vi "EnumDevicesByGenTL.vi"(0 "error in (no error)":errorcluster caption="错误输入（无错误）", 1 "pIFInfo":T2) -> (2 "error out":errorcluster caption="错误输出", 3 "function return":i32, 4 "nDeviceNum":u32, 5 "pGenTLDevInfoArray":T1(array[cluster]))   [LabVIEW 2013, in "MvCameraControl.lvlib"]
uses:
  MvCameraControl.lvlib
  MvCameraPatch.dll
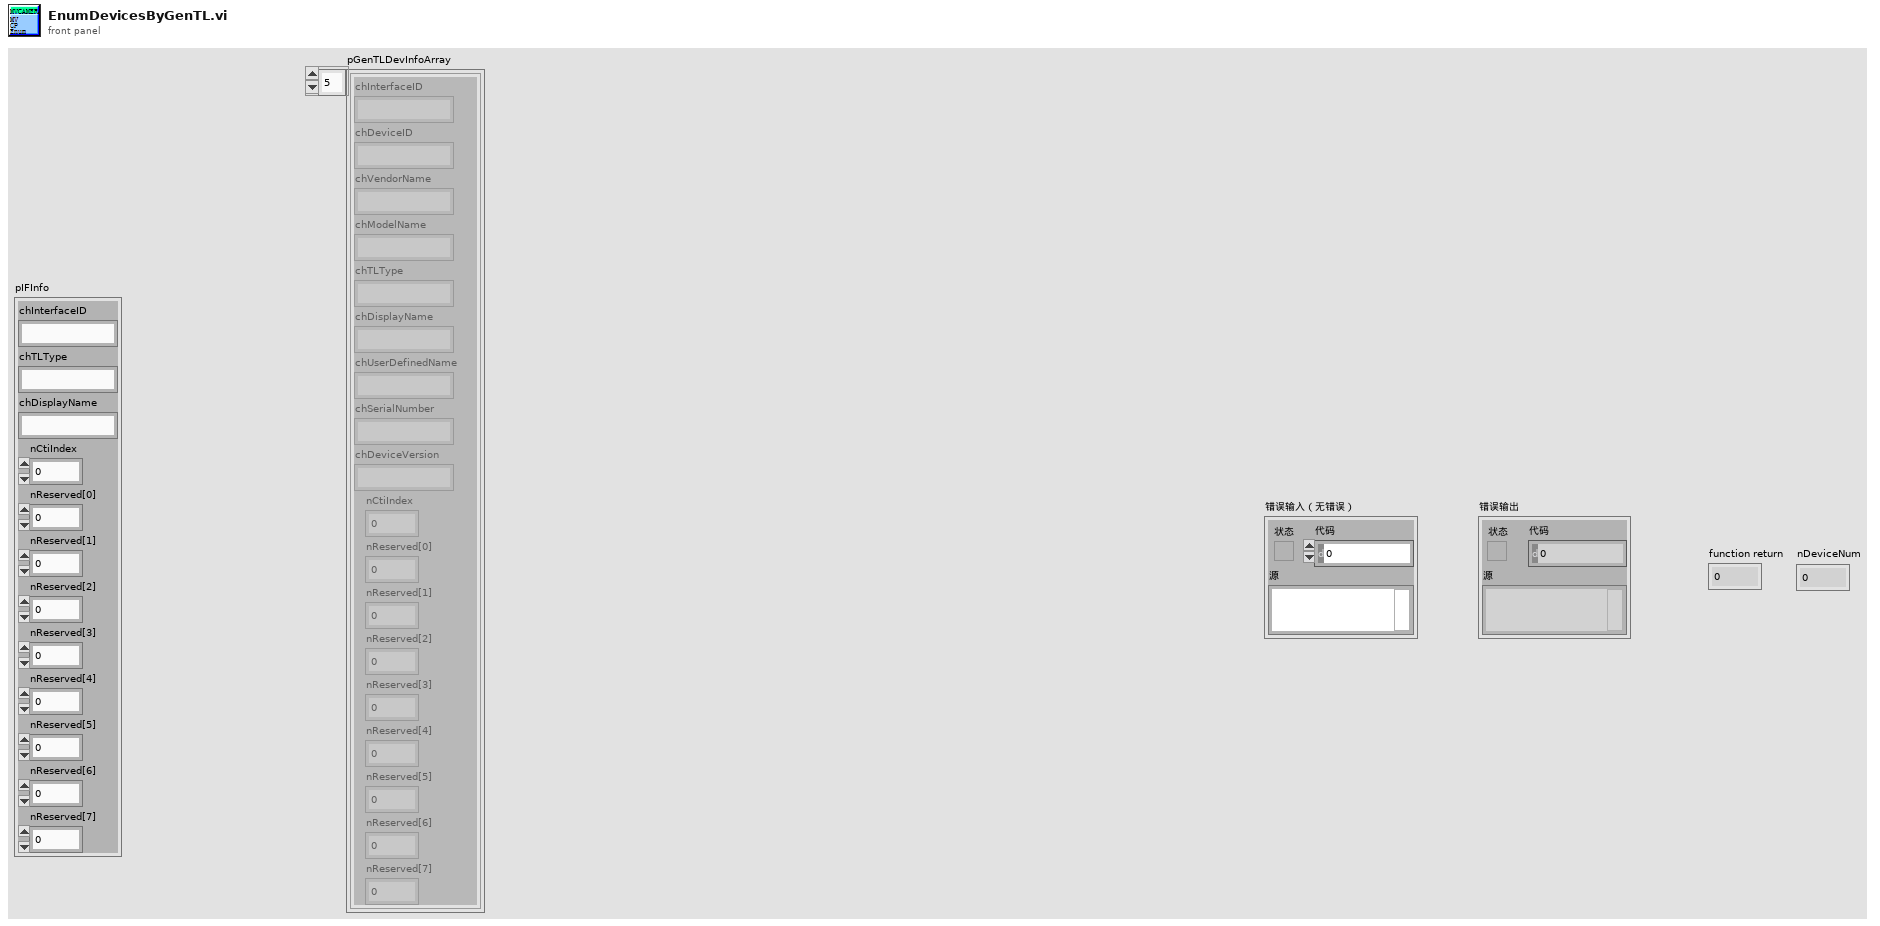
[diagram p1: front panel]
types:
  T1 = cluster{"chInterfaceID":string, "chDeviceID":string, "chVendorName":string, "chModelName":string, "chTLType":string, "chDisplayName":string, "chUserDefinedName":string, "chSerialNumber":string, "chDeviceVersion":string, "nCtiIndex":u32, "nReserved[0]":u32, "nReserved[1]":u32, "nReserved[2]":u32, "nReserved[3]":u32, "nReserved[4]":u32, "nReserved[5]":u32, "nReserved[6]":u32, "nReserved[7]":u32}[]
  T2 = cluster{"chInterfaceID":string, "chTLType":string, "chDisplayName":string, "nCtiIndex":u32, "nReserved[0]":u32, "nReserved[1]":u32, "nReserved[2]":u32, "nReserved[3]":u32, "nReserved[4]":u32, "nReserved[5]":u32, "nReserved[6]":u32, "nReserved[7]":u32}
  T3 = cluster{"chInterfaceID":string, "chDeviceID":string, "chVendorName":string, "chModelName":string, "chTLType":string, "chDisplayName":string, "chUserDefinedName":string, "chSerialNumber":string, "chDeviceVersion":string, "nCtiIndex":u32, "nReserved[0]":u32, "nReserved[1]":u32, "nReserved[2]":u32, "nReserved[3]":u32, "nReserved[4]":u32, "nReserved[5]":u32, "nReserved[6]":u32, "nReserved[7]":u32}
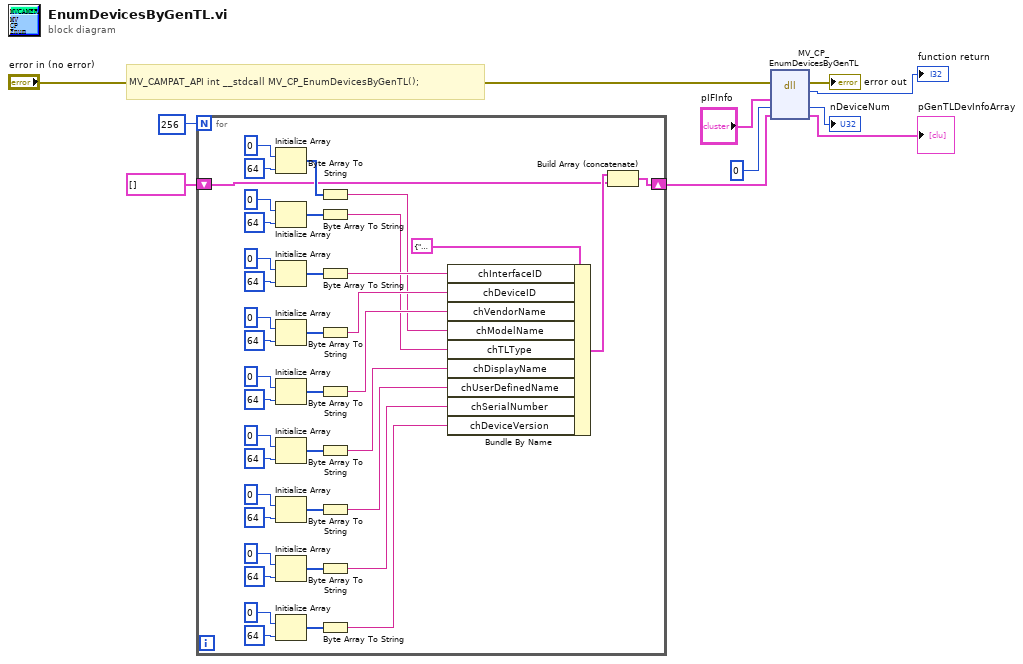
[diagram p0: block diagram]
diagram:
  # "MV_CAMPAT_API int __stdcall MV_CP_EnumDevicesByGenTL();"
  n1 = for {
    N: 256 -> [_]
    shift-right: [w12] -> w2
    shift-left: T1 [] ("pDeviceInfoTemp") -> [w11]
    n2 = Initialize Array(u8 0 ("元素"), 64 ("维数大小")) -> (w40:u8[])
    n3 = Initialize Array(u8 0 ("元素"), 64 ("维数大小")) -> (w37:u8[])
    n4 = Initialize Array(u8 0 ("元素"), 64 ("维数大小")) -> (w50:u8[])
    n5 = Initialize Array(u8 0 ("元素"), 64 ("维数大小")) -> (w46:u8[])
    n6 = Initialize Array(u8 0 ("元素"), 64 ("维数大小")) -> (w21:u8[])
    n7 = Initialize Array(u8 0 ("元素"), 64 ("维数大小")) -> (w34:u8[])
    n8 = Initialize Array(u8 0 ("元素"), 64 ("维数大小")) -> (w31:u8[])
    n9 = Initialize Array(u8 0 ("元素"), 64 ("维数大小")) -> (w19:u8[])
    n10 = Initialize Array(u8 0 ("元素"), 64 ("维数大小")) -> (w26:u8[])
    n11 = Byte Array To String(unsigned byte array=w40) -> (string=w17:string)
    n12 = Byte Array To String(unsigned byte array=w37) -> (string=w22:string)
    n13 = Byte Array To String(unsigned byte array=w50) -> (string=w47:string)
    n14 = Byte Array To String(unsigned byte array=w46) -> (string=w43:string)
    n15 = Byte Array To String(unsigned byte array=w21) -> (string=w23:string)
    n16 = Byte Array To String(unsigned byte array=w34) -> (string=w20:string)
    n17 = Byte Array To String(unsigned byte array=w31) -> (string=w16:string)
    n18 = Byte Array To String(unsigned byte array=w19) -> (string=w15:string)
    n19 = Byte Array To String(unsigned byte array=w26) -> (string=w14:string)
    n20 = Bundle By Name(cluster=T3 {"chInterfaceID"="", "chDeviceID"="", "chVendorName"="", "chModelName"="", "chTLType"="", "chDisplayName"="", "chUserDefinedName"="", "chSerialNumber"="", "chDeviceVersion"="", "nCtiIndex"=0, "nReserved[0]"=0, "nReserved[1]"=0, "nReserved[2]"=0, "nReserved[3]"=0, "nReserved[4]"=0, "nReserved[5]"=0, "nReserved[6]"=0, "nReserved[7]"=0} ("pDeviceInfo 2"), "chInterfaceID"=w47, "chDeviceID"=w43, "chVendorName"=w23, "chModelName"=w17, "chTLType"=w22, "chDisplayName"=w20, "chUserDefinedName"=w16, "chSerialNumber"=w15, "chDeviceVersion"=w14) -> (w18:T3)
    n21 = Build Array (concatenate)(w18, w11) -> (w12:T1)
  }
  n22 = dll-call lib="MvCameraPatch.dll" fn="MV_CP_EnumDevicesByGenTL"(error in="error in (no error)", "pstIFInfo"="pIFInfo", "nDeviceNum"=u32 0, "pGenTLDevInfoArray"=w2) -> (error out=→"error out":errorcluster, "返回类型"=→"function return":i32, "nDeviceNum"=→"nDeviceNum":u32, "pGenTLDevInfoArray"=→"pGenTLDevInfoArray":T1)  [unwired: 3 in, 1 out]
